vi "Project.vi"() -> ()   [LabVIEW 2022 SP3]
uses:
  <vilib>/DAQmx/read.llb/DAQmx Read (Digital Bool 1Line 1Point).vi
  <vilib>/DAQmx/write.llb/DAQmx Write (Digital Bool 1Line 1Point).vi
  <vilib>/DAQmx/read.llb/DAQmx Read (Analog DBL 1Chan 1Samp).vi
  <vilib>/DAQmx/create/channels.llb/DAQmx Create Channel (DO-Digital Output).vi
  <vilib>/DAQmx/miscellaneous.llb/DAQmx Fill In Error Info.vi
  <vilib>/DAQmx/create/channels.llb/DAQmx Create Channel (AI-Voltage-Basic).vi
  <vilib>/DAQmx/configure/timing.llb/DAQmx Timing (Sample Clock).vi
  <vilib>/DAQmx/create/channels.llb/DAQmx Create Channel (DI-Digital Input).vi
  <vilib>/httpClient/LabVIEWHTTPClient.lvlib
panel:
  out "PIR":bool
  in  "stop 2":bool
  in  "PIR output to pi":tag
  in  "PIR input":tag
  in  "stop":bool
  in  "DAQmx Physical Channel 4":tag
  in  "Sampling Frequency LDR":dbl
  in  "DAQmx Physical Channel 3":tag
  in  "DAQmx Physical Channel":tag
  out "String 2":string
  out "Cluster 2":T1
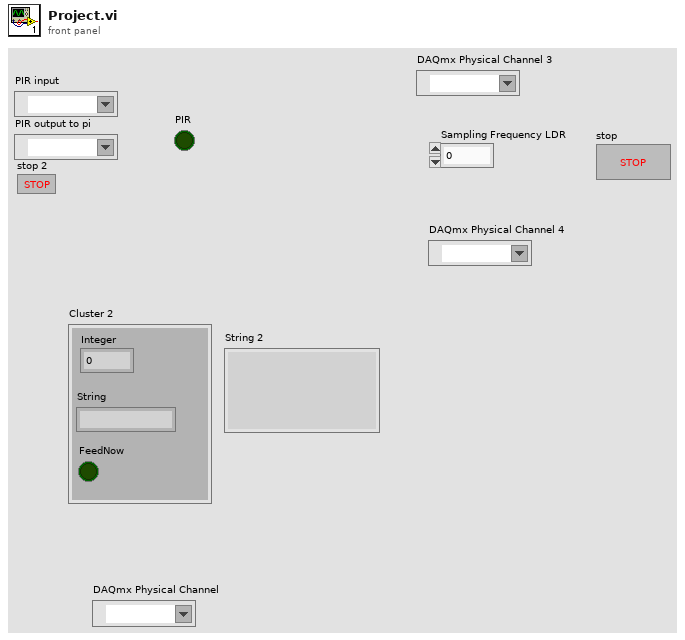
[diagram p1: front panel]
types:
  T1 = cluster{"Integer":dbl, "String":string, "FeedNow":bool}
  T2 = cluster{"Integer":i32, "String":string, "FeedNow":bool}
  T3 = typedef "LabVIEWHTTPClient.lvlib/ClientHandle.ctl" = refnum<k1>
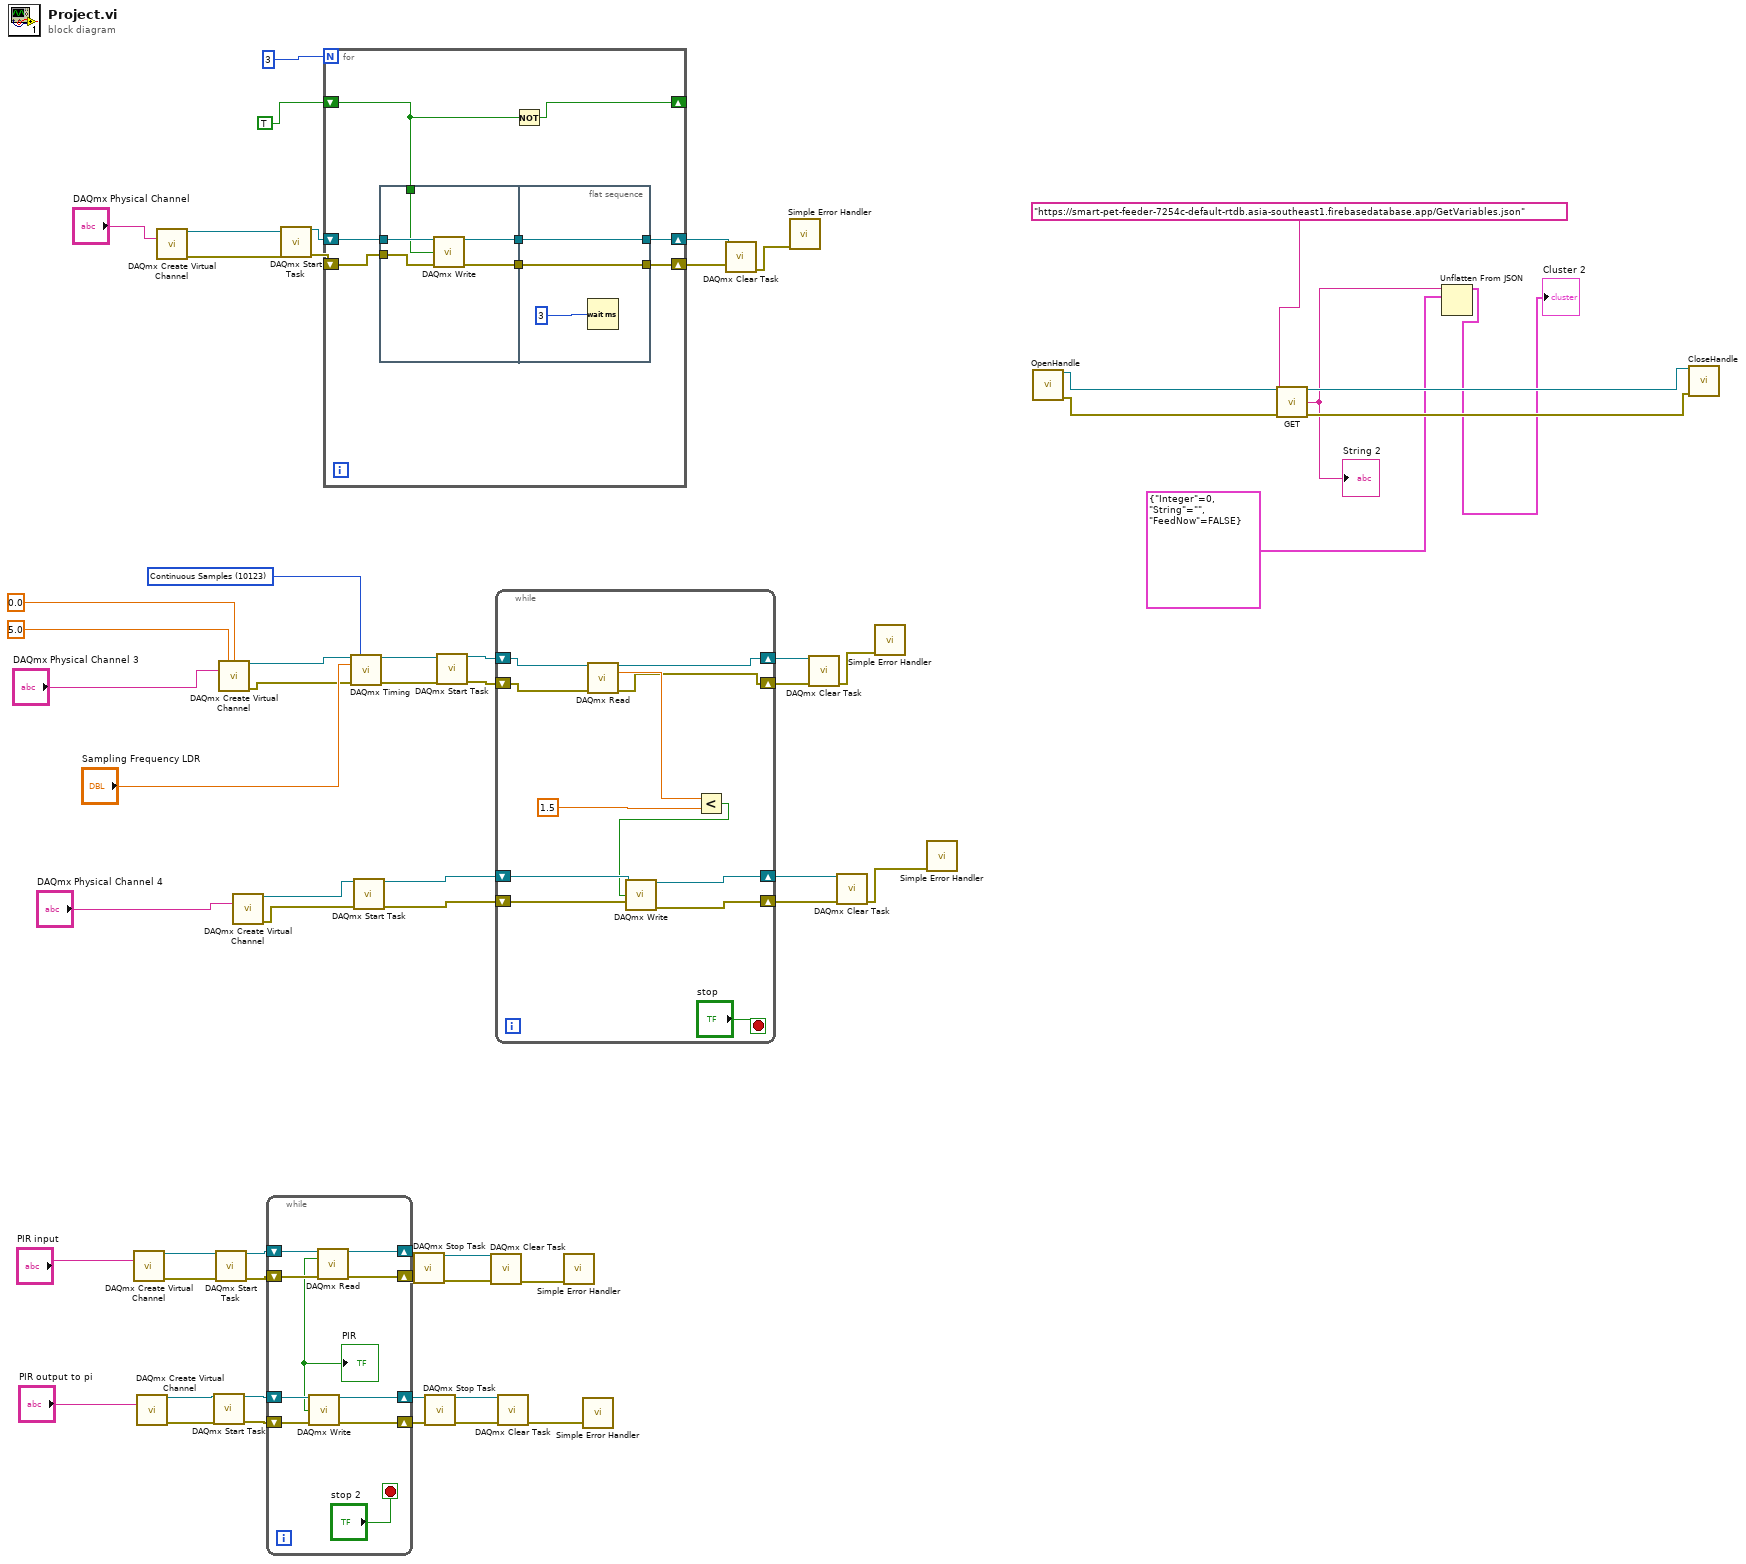
[diagram p0: block diagram]
diagram:
  w39 = 10123 items=["Finite Samples"=10178, "Continuous Samples"=10123, "Hardware Timed Single Point"=12522] ("sample mode")
  n1 = call-poly <vilib>:"DAQmx Create Virtual Channel.vi"("lines"="PIR input") -> ("task out"=w19:refnum<k21>, "error out"=w18:errorcluster)  [unwired: 13 in]
  n2 = call-poly <vilib>:"DAQmx Create Virtual Channel.vi"("lines"="PIR output to pi") -> ("task out"=w13:refnum<k21>, "error out"=w12:errorcluster)  [unwired: 13 in]
  n3 = call-poly <vilib>:"DAQmx Create Virtual Channel.vi"("lines"="DAQmx Physical Channel") -> ("task out"=w53:refnum<k21>, "error out"=w51:errorcluster)  [unwired: 13 in]
  n4 = call <vilib>:"DAQmx Start Task.vi"("task/channels in"=w13, "error in"=w12) -> ("task out"=w4:refnum<k21>, "error out"=w2:errorcluster)  [unwired: 12 in]
  n5 = call <vilib>:"DAQmx Start Task.vi"("task/channels in"=w19, "error in"=w18) -> ("task out"=w8:refnum<k21>, "error out"=w5:errorcluster)  [unwired: 12 in]
  n6 = call-poly <vilib>:"DAQmx Create Virtual Channel.vi"("maximum value"=5.0, "minimum value"=0.0, "physical channels"="DAQmx Physical Channel 3") -> ("task out"=w38:refnum<k21>, "error out"=w36:errorcluster)  [unwired: 11 in]
  n7 = call-poly <vilib>:"DAQmx Create Virtual Channel.vi"("lines"="DAQmx Physical Channel 4") -> ("task out"=w31:refnum<k21>, "error out"=w30:errorcluster)  [unwired: 13 in]
  n8 = while {
    shift-right: [w69] -> w7
    shift-left: w8 -> [w70]
    shift-right: [w68] -> w6
    shift-left: w5 -> [w67]
    shift-right: [w65] -> w3
    shift-left: w4 -> [w66]
    shift-right: [w63] -> w1
    shift-left: w2 -> [w64]
    stop <- "stop 2" stop-if-true
    n9 = call-poly <vilib>:"DAQmx Read.vi"("task/channels in"=w70, "error in"=w67) -> ("task out"=w69:refnum<k21>, "data"=w61:bool, "error out"=w68:errorcluster)  [unwired: 11 in]
    "PIR" <- w61
    n10 = call-poly <vilib>:"DAQmx Write.vi"("task/channels in"=w66, "data"=w61, "error in"=w64) -> ("task out"=w65:refnum<k21>, "error out"=w63:errorcluster)  [unwired: 10 in, 1 out]
  }
  n11 = call <vilib>:"DAQmx Start Task.vi"("task/channels in"=w53, "error in"=w51) -> ("task out"=w52:refnum<k21>, "error out"=w50:errorcluster)  [unwired: 12 in]
  n12 = for {
    N: 3 -> [_]
    shift-right: [w74] -> w48
    shift-left: w52 -> [w76]
    shift-right: [w73] -> w47
    shift-left: w50 -> [w75]
    shift-right: [w71] -> _
    shift-left: TRUE -> [w72]
    n13 = flat-sequence {
      tunnel: w76 -> [w83]
      tunnel: w75 -> [w82]
      tunnel: [w81] -> w78
      tunnel: [w80] -> w77
      tunnel: w72 -> [w79]
      tunnel: w78 -> [w85]
      tunnel: [w85] -> w74
      tunnel: [w84] -> w73
      tunnel: w77 -> [w84]
      frame #0 {
        n14 = call-poly <vilib>:"DAQmx Write.vi"("task/channels in"=w83, "data"=w79, "error in"=w82) -> ("task out"=w81:refnum<k21>, "error out"=w80:errorcluster)  [unwired: 10 in, 1 out]
      }
      frame #1 {
        n15 = Wait (ms)(milliseconds to wait=u32 3) -> ()  [unwired: 1 out]
      }
    }
    n16 = Not(x=w72) -> (.not. x?=w71:bool)
  }
  n17 = call-poly <vilib>:"DAQmx Timing.vi"("task/channels in"=w38, "sample mode"=w39, "rate"="Sampling Frequency LDR", "error in"=w36) -> ("task out"=w37:refnum<k21>, "error out"=w35:errorcluster)  [unwired: 10 in]
  n18 = call <vilib>:"DAQmx Start Task.vi"("task/channels in"=w31, "error in"=w30) -> ("task out"=w29:refnum<k21>, "error out"=w22:errorcluster)  [unwired: 12 in]
  n19 = call <vilib>:"DAQmx Stop Task.vi"("task/channels in"=w7, "error in"=w6) -> ("task out"=w17:refnum<k21>, "error out"=w16:errorcluster)  [unwired: 12 in]
  n20 = call <vilib>:"DAQmx Stop Task.vi"("task/channels in"=w3, "error in"=w1) -> ("task out"=w11:refnum<k21>, "error out"=w10:errorcluster)  [unwired: 12 in]
  n21 = call <vilib>:"DAQmx Start Task.vi"("task/channels in"=w37, "error in"=w35) -> ("task out"=w34:refnum<k21>, "error out"=w33:errorcluster)  [unwired: 12 in]
  n22 = call <vilib>:"DAQmx Clear Task.vi"("task in"=w17, "error in"=w16) -> ("error out"=w15:errorcluster)  [unwired: 13 in]
  n23 = while {
    shift-right: [w92] -> w28
    shift-left: w34 -> [w98]
    shift-right: [w91] -> w27
    shift-left: w33 -> [w97]
    shift-right: [w90] -> w24
    shift-left: w29 -> [w95]
    shift-right: [w89] -> w23
    shift-left: w22 -> [w88]
    stop <- "stop" stop-if-true
    n24 = call-poly <vilib>:"DAQmx Read.vi"("task/channels in"=w98, "error in"=w97) -> ("task out"=w92:refnum<k21>, "data"=w94:dbl, "error out"=w91:errorcluster)  [unwired: 11 in]
    n25 = Less?(x=w94, y=1.5) -> (x < y?=w93:bool)
    n26 = call-poly <vilib>:"DAQmx Write.vi"("task/channels in"=w95, "data"=w93, "error in"=w88) -> ("task out"=w90:refnum<k21>, "error out"=w89:errorcluster)  [unwired: 10 in, 1 out]
  }
  n27 = call <vilib>:"DAQmx Clear Task.vi"("task in"=w11, "error in"=w10) -> ("error out"=w9:errorcluster)  [unwired: 13 in]
  n28 = call <vilib>:"Simple Error Handler.vi"("error in (no error)"=w15) -> ()  [unwired: 4 in, 5 out]
  n29 = call <vilib>:"Simple Error Handler.vi"("error in (no error)"=w9) -> ()  [unwired: 4 in, 5 out]
  n30 = call <vilib>:"DAQmx Clear Task.vi"("task in"=w48, "error in"=w47) -> ("error out"=w46:errorcluster)  [unwired: 13 in]
  n31 = call <vilib>:"Simple Error Handler.vi"("error in (no error)"=w46) -> ()  [unwired: 4 in, 5 out]
  n32 = call <vilib>:"DAQmx Clear Task.vi"("task in"=w28, "error in"=w27) -> ("error out"=w26:errorcluster)  [unwired: 13 in]
  n33 = call <vilib>:"DAQmx Clear Task.vi"("task in"=w24, "error in"=w23) -> ("error out"=w25:errorcluster)  [unwired: 13 in]
  n34 = call <vilib>:"Simple Error Handler.vi"("error in (no error)"=w26) -> ()  [unwired: 4 in, 5 out]
  n35 = call <vilib>:"Simple Error Handler.vi"("error in (no error)"=w25) -> ()  [unwired: 4 in, 5 out]
  n36 = call <vilib>:"OpenHandle.vi"() -> ("client handle out"=w59:T3, "error out"=w57:errorcluster)  [unwired: 14 in]
  n37 = call <vilib>:"GET.vi"("client handle"=w59, "url"="https://smart-pet-feeder-7254c-default-rtdb.asia-southeast1.firebasedatabase.app/GetVariables.json", "error in (no error)"=w57) -> ("client handle out"=w58:T3, "body"=w55:string, "error out"=w56:errorcluster)  [unwired: 9 in, 1 out]
  "String 2" <- w55
  n38 = Unflatten From JSON(JSON string=w55, type and defaults=T2 {"Integer"=0, "String"="", "FeedNow"=FALSE}) -> (value=→"Cluster 2":T2)  [unwired: 5 in, 1 out]
  n39 = call <vilib>:"CloseHandle.vi"("client handle"=w58, "error in (no error)"=w56) -> ()  [unwired: 13 in, 1 out]
